vi "HexStringToHexDisplayString.vi"(11 "正常显示HEX字符串":string) -> (3 "HEX显示字符串":string)   [LabVIEW 2015, in "WZ5005E.lvlib"]
uses:
  WZ5005E.lvlib
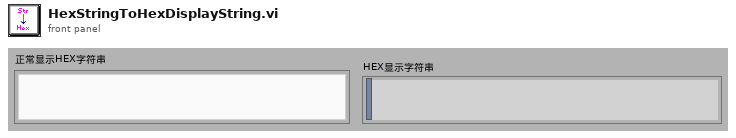
[diagram p1: front panel]
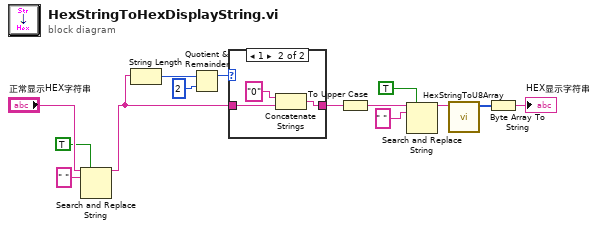
[diagram p0: block diagram]
diagram:
  n1 = Search and Replace String(replace all?=TRUE ("替换全部？(F)"), input string="正常显示HEX字符串", search string=" " ("搜索字符串")) -> (result string=w3:string)  [unwired: 5 in, 3 out]
  n2 = String Length(string=w3) -> (length=w8:i32)
  n3 = Quotient & Remainder(x=w8, y=2) -> (x-y*floor(x/y)=w6:i32)  [unwired: 1 out]
  n4 = case shown="1" w6 {
    tunnel: w3 -> [w15 w18]
    tunnel: [w15 w16] -> w5
    frame 0, Default {
    }
    frame 1 {
      n5 = Concatenate Strings("0" ("字符串"), w18) -> (w16:string)
    }
  }
  n6 = To Upper Case(1:w5) -> (0:w9:string)
  n7 = Search and Replace String(replace all?=TRUE ("替换全部？(F)"), input string=w9, search string=" " ("搜索字符串")) -> (result string=w12:string)  [unwired: 5 in, 3 out]
  n8 = call "HexStringToU8Array.vi"("HEX String (0-9,A-F)"=w12) -> ("u8 Data[]"=w14:u8[])  [unwired: 10 in]
  n9 = Byte Array To String(unsigned byte array=w14) -> (string=→"HEX显示字符串":string)
